vi "Manlight - Query Error.vi"(8 "error in (no error)":errorcluster, 11 "VISA Refnum in":refnum<visa-resource-name>) -> (0 "error out":errorcluster, 2 "Error Status":string, 3 "VISA Refnum out":refnum<visa-resource-name>)   [LabVIEW 2020]
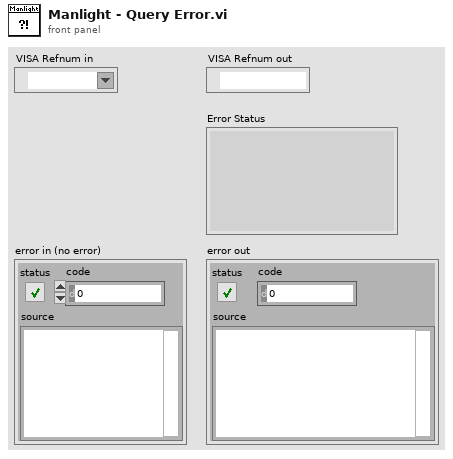
[diagram p1: front panel]
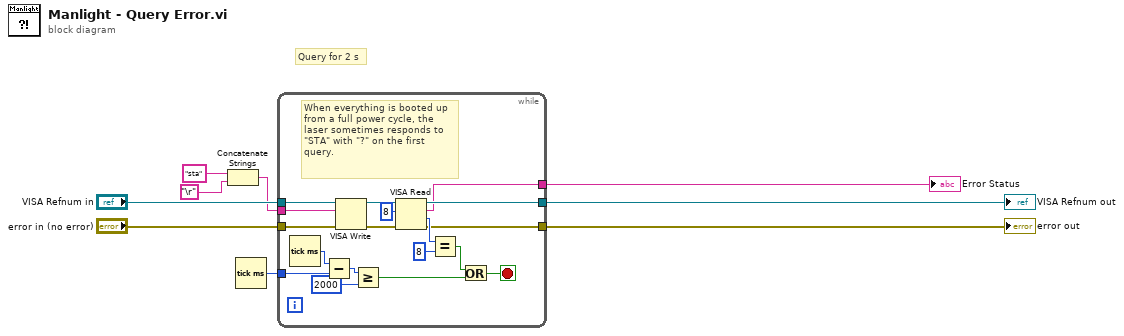
[diagram p0: block diagram]
diagram:
  # "Query for 2 s"
  n1 = Concatenate Strings("sta", "\r") -> (w5:string)
  n2 = Tick Count (ms)() -> (millisecond timer value=w1:u32)
  n3 = while {
    tunnel: w5 -> [w25]
    tunnel: "VISA Refnum in" -> [w26]
    tunnel: "error in (no error)" -> [w27]
    tunnel: [w19] -> w4
    tunnel: [w18] -> w3
    tunnel: [w17] -> w2
    tunnel: w1 -> [w14]
    stop <- w11 stop-if-true
    # "When everything is booted up from a full power cycle, the laser sometimes responds to \"STA\" with \"?\" on the first query."
    n4 = Tick Count (ms)() -> (millisecond timer value=w15:u32)
    n5 = Subtract(x=w15, y=w14) -> (x-y=w13:u32)
    n6 = VISA Write(VISA resource name=w26, write buffer=w25, error in (no error)=w27) -> (VISA resource name out=w21:refnum<visa-resource-name>, error out=w22:errorcluster)  [unwired: 1 out]
    n7 = Greater Or Equal?(x=w13, y=u32 2000) -> (x >= y?=w10:bool)
    n8 = VISA Read(VISA resource name=w21, byte count=u32 8, error in (no error)=w22) -> (VISA resource name out=w19:refnum<visa-resource-name>, read buffer=w17:string, return count=w20:u32, error out=w18:errorcluster)
    n9 = Equal?(x=w20, y=u32 8) -> (x = y?=w16:bool)
    n10 = Or(x=w16, y=w10) -> (x .or. y?=w11:bool)
  }
  "error out" <- w3
  "Error Status" <- w2
  "VISA Refnum out" <- w4
